vi "ziExample-ListDevices.vi"() -> ()   [LabVIEW 2009]
doc: "Control a Zurich instrument device via the LabOne Labview API. \nRequirements: Zurich Instruments MFLI, HF2 or UHFLI \nThis is an example for the Zurich Instruments LabOne LabVIEW API. This example lists all available instruments and displays some information on them.\n\n© Zurich Instruments AG, www.zhinst.com"
uses:
  <instrlib>/Zurich Instruments LabOne/Public/ziTypeDisovery.ctl
  <instrlib>/Zurich Instruments LabOne/Zurich Instruments LabOne.lvlib
panel:
  in  "Connect":bool
  out "Connected Device":string
  out "Error Out":errorcluster
  out "ziDiscovery":T1={"timestamp"=0, "deviceid"="", "devicetype"="", "serveraddress"="", "serverport"=0, "apilevel"=0, "discoverable"=TRUE, "interface"="", "connected"="", "available"=TRUE, "owner"="", "status"="", "options "="", "serverversion"=""}
  in  "stop":bool
  in  "Listbox":i32(listbox)
  # "ziExample-ListDevices.vi\nRequirements: HF2LI, UHFLI or MFLI\nsee block diagram for VI description"
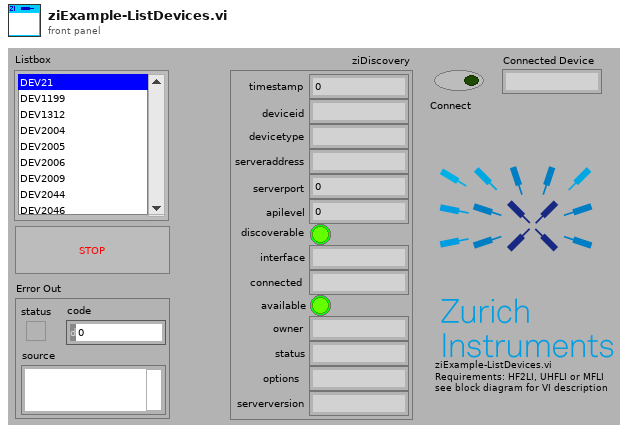
[diagram p1: front panel]
types:
  T1 = typedef "ziTypeDisovery.ctl" = cluster{"timestamp":u64, "deviceid":string, "devicetype":string, "serveraddress":string, "serverport":u32, "apilevel":u32, "discoverable":bool, "interface":string, "connected":string, "available":bool, "owner":string, "status":string, "options ":string, "serverversion":string}
  T2 = typedef "Zurich Instruments LabOne.lvlib/ziTypeHandle.ctl" = cluster{"handleValid":bool, "Conn":u64, "Path Prefix":string, "Handle":u64, "Connected":bool, "Clockbase(s)":dbl}
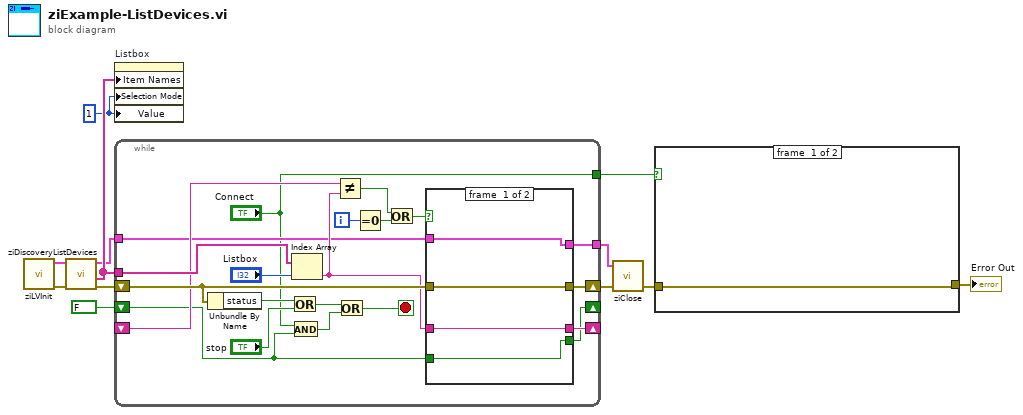
[diagram p0: block diagram]
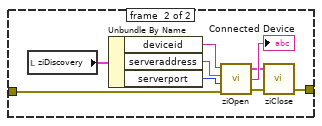
[diagram p2: hidden frame]
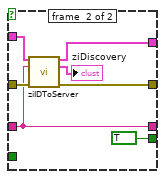
[diagram p3: hidden frame]
diagram:
  w8 = 1 ("Selection Mode")
  n1 = call <instrlib>:"ziLVInit.vi"() -> ("Error Out"=w12:errorcluster, "ziHandle"=w7:T2)  [unwired: 10 in]
  n2 = call <instrlib>:"ziDiscoveryListDevices.vi"("Error In"=w12, "ziHandle In"=w7) -> ("Error Out"=w10:errorcluster, "DevicesList"=w11:string[], "ziHandle Out"=w6:T2)  [unwired: 7 in]
  n3 = property on="Listbox" class="LstBox (strict)"("Item Names"=w11, "Selection Mode"=w8, "Value"=w8) -> ()  [unwired: 2 in, 2 out]
  n4 = while {
    tunnel: w11 -> [w32]
    shift-right: [w33] -> w9
    shift-left: w10 -> [w31]
    shift-right: [w28] -> _
    shift-left: _ -> [w26]
    tunnel: w6 -> [w21]
    tunnel: [w20] -> w5
    shift-right: [w18] -> _
    shift-left: FALSE -> [w17]
    tunnel: ["Connect"] -> w3
    i -> [w25]
    stop <- w15 stop-if-true
    n5 = Unbundle By Name(w31) -> ("status"=w30:bool)
    n6 = Or(x=w30, y="stop") -> (x .or. y?=w16:bool)
    n7 = And(x="Connect", y=w17) -> (x .and. y?=w14:bool)
    n8 = Index Array(array=w32, index="Listbox") -> (element=w27:string)
    n9 = Not Equal?(x=w26, y=w27) -> (x != y?=w24:bool)
    n10 = Or(x=w16, y=w14) -> (x .or. y?=w15:bool)
    n11 = Equal To 0?(x=w25) -> (x = 0?=w23:bool)
    n12 = Or(x=w24, y=w23) -> (x .or. y?=w22:bool)
    n13 = case shown="True" w22 {
      tunnel: [w36 w44] -> w33
      tunnel: w27 -> [w37 w41]
      tunnel: w31 -> [w36 w43]
      tunnel: [w37 w41] -> w28
      tunnel: w21 -> [w35 w40]
      tunnel: [w35 w39] -> w20
      tunnel: w17 -> [w34 _]
      tunnel: [w34 TRUE] -> w18
      frame #0 {
      }
      frame #1 {
        n14 = call <instrlib>:"ziIDToServer.vi"("ziHandle In"=w40, "Device ID"=w41, "Error In"=w43) -> ("ziHandle Out"=w39:T2, "ziDiscovery"=→"ziDiscovery":T1, "Error Out"=w44:errorcluster)  [unwired: 10 in]
      }
    }
  }
  n15 = call <instrlib>:"ziClose.vi"("Error In"=w9, "Handle In"=w5) -> ("Error Out"=w1:errorcluster)  [unwired: 2 in, 1 out]
  n16 = case shown="False" w3 {
    tunnel: [w45 w50] -> w2
    tunnel: w1 -> [w45 w49]
    frame #0 {
    }
    frame #1 {
      n17 = local read "ziDiscovery"() -> (w51:T1)
      n18 = Unbundle By Name(w51) -> ("deviceid"=w48:string, "serveraddress"=w47:string, "serverport"=w46:u32)
      n19 = call <instrlib>:"ziOpen.vi"("Error In"=w49, "Port obsolete (auto)"=w46, "Hostname obsolete (auto)"=w47, "Address"=w48) -> ("Error Out"=w52:errorcluster, "Selected Device"=→"Connected Device":string, "HandleOut"=w53:T2)
      n20 = call <instrlib>:"ziClose.vi"("Error In"=w52, "Handle In"=w53) -> ("Error Out"=w50:errorcluster)  [unwired: 2 in, 1 out]
    }
  }
  "Error Out" <- w2
